vi "Init DMM - Voltage Mode.vi"(8 "error in (no error)":errorcluster, 9 "Switch -> DMM Trigger":u16, 10 "DMM -> Switch Trigger":u16, 11 "DMM Device in":refnum<k15>) -> (0 "error out":errorcluster, 3 "DMM Device out":refnum<k15>)   [LabVIEW 2011, in "Switch-DMM Custom Device.lvlib"]
uses:
  Switch-DMM Custom Device.lvlib
  <instrlib>/niDMM/nidmm.llb/niDMM Resolution in Digits.ctl
  <instrlib>/niDMM/nidmm.llb/niDMM Slope.ctl
  <instrlib>/niDMM/nidmm.llb/niDMM Sample Trigger.ctl
  <instrlib>/niDMM/nidmm.llb/niDMM Trigger.ctl
  <instrlib>/niDMM/nidmm.llb/niDMM Measurement Complete.ctl
  <instrlib>/niDMM/nidmm.llb/niDMM Function.ctl
  <instrlib>/niDMM/nidmm.llb/niDMM Configure Measurement Digits.vi
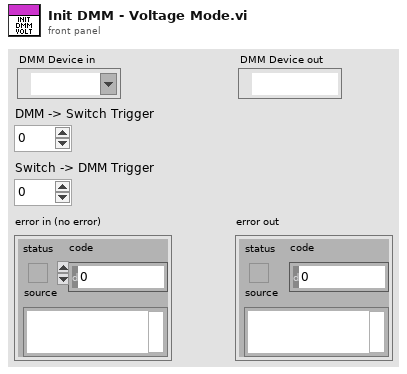
[diagram p1: front panel]
types:
  T1 = typedef "niDMM Sample Trigger.ctl" = enum16{"Immediate", "External", "TTL 0", "TTL 1", "TTL 2", "TTL 3", "TTL 4", "TTL 5", "TTL 6", "Interval", "Software", "TTL 7", "PXI Star", "LBR Trig 1", "Aux Trig 1"}
  T2 = typedef "niDMM Trigger.ctl" = enum16{"Immediate", "External", "TTL 0", "TTL 1", "TTL 2", "TTL 3", "TTL 4", "TTL 5", "TTL 6", "Software", "TTL 7", "PXI Star", "LBR Trig 1", "Aux Trig 1"}
  T3 = typedef "niDMM Measurement Complete.ctl" = enum16{"None", "External", "TTL 0", "TTL 1", "TTL 2", "TTL 3", "TTL 4", "TTL 5", "TTL 6", "TTL 7", "LBR Trig 0"}
  T4 = typedef "niDMM Function.ctl" = enum16{"DC Volts", "AC Volts", "DC Current", "AC Current", "2-wire Resistance", "4-wire Resistance", "Diode", "Frequency", "Period", "AC Volts DC Coupled", "Capacitance", "Inductance", "Temperature"}
  T5 = typedef "niDMM Resolution in Digits.ctl" = dbl
  T6 = typedef "niDMM Slope.ctl" = enum16{"Rising Edge", "Falling Edge"}
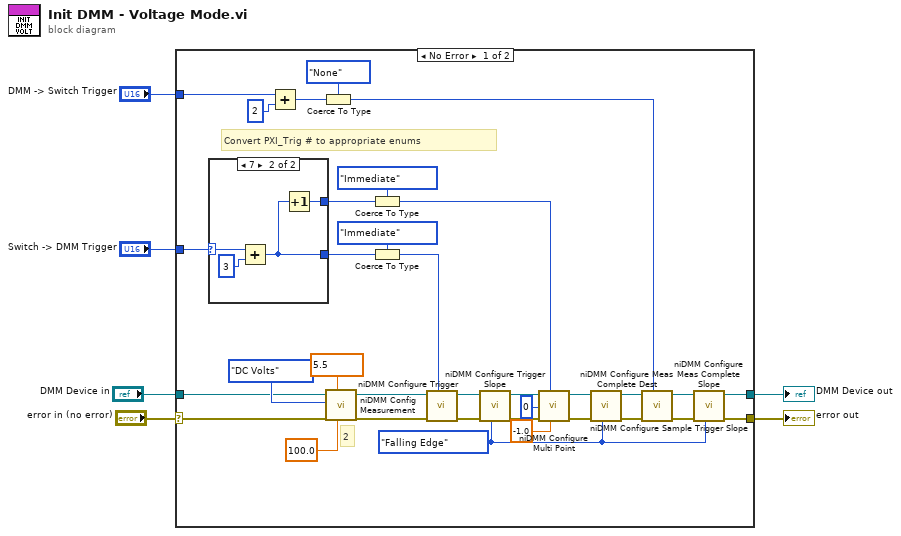
[diagram p0: block diagram]
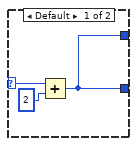
[diagram p2: hidden frame]
diagram:
  n1 = case shown="No Error" "error in (no error)" {
    selector: "error in (no error)" -> [w10 w48]
    tunnel: [w40 w49] -> w1
    tunnel: [w39 w48] -> w2
    tunnel: "DMM Device in" -> [w11 w49]
    tunnel: "DMM -> Switch Trigger" -> [w20 _]
    tunnel: "Switch -> DMM Trigger" -> [w18 _]
    frame No Error {
      w7 = T5 5.5 items=["3 1/2"=3.5, "4 1/2"=4.5, "5 1/2"=5.5, "6 1/2"=6.5, "7 1/2"=7.5] ("Resolution in Digits")
      w9 = niDMM_Slope."Falling Edge" ("Slope")
      # "Convert PXI_Trig # to appropriate enums"
      # "2"
      n2 = case shown="7" w18 {
        selector: w18 -> [w42 w46]
        tunnel: [w41 w45] -> w17
        tunnel: [w41 w44] -> w14
        frame Default {
          n3 = Add(x=w42, y=u16 2) -> (x+y=w41:u16)
        }
        frame 7 {
          n4 = Add(x=w46, y=u16 3) -> (x+y=w45:u16)
          n5 = Increment(x=w45) -> (x+1=w44:u16)
        }
      }
      n6 = Add(x=w20, y=u16 2) -> (x+y=w22:u16)
      n7 = Coerce To Type(0:w22, 1:niDMM_Measurement_Complete."None" ("Measurement Complete Destination")) -> (2:w19:T3)
      n8 = call-poly <instrlib>:"niDMM Config Measurement.vi"("Range"=100.0 ("range"), "Resolution in Digits"=w7, "error in (no error)"=w10, "Function"=niDMM_Function."DC Volts" ("measurement type"), "instrument handle"=w11) -> ("error out"=w24:errorcluster, "instrument handle out"=w25:refnum<k15>)  [unwired: 5 out]
      n9 = Coerce To Type(0:w14, 1:niDMM_Sample_Trigger."Immediate" ("Sample Trigger")) -> (2:w12:T1)
      n10 = Coerce To Type(0:w17, 1:niDMM_Trigger."Immediate" ("trigger source")) -> (2:w15:T2)
      n11 = call <instrlib>:"niDMM Configure Trigger.vi"("Trigger Source"=w15, "error in (no error)"=w24, "instrument handle"=w25) -> ("error out"=w37:errorcluster, "instrument handle out"=w38:refnum<k15>)  [unwired: 1 in, 6 out]
      n12 = call <instrlib>:"niDMM Configure Trigger Slope.vi"("Slope"=w9, "error in (no error)"=w37, "instrument handle"=w38) -> ("error out"=w35:errorcluster, "instrument handle out"=w36:refnum<k15>)  [unwired: 7 out]
      n13 = call <instrlib>:"niDMM Configure Multi Point.vi"("Sample Interval (sec)"=-1.0, "Sample Trigger"=w12, "error in (no error)"=w35, "Sample Count"=0 ("sample count"), "instrument handle"=w36) -> ("error out"=w33:errorcluster, "instrument handle out"=w34:refnum<k15>)  [unwired: 1 in, 4 out]
      n14 = call <instrlib>:"niDMM Configure Sample Trigger Slope.vi"("Slope"=w9, "error in (no error)"=w33, "instrument handle"=w34) -> ("error out"=w31:errorcluster, "instrument handle out"=w30:refnum<k15>)  [unwired: 7 out]
      n15 = call <instrlib>:"niDMM Configure Meas Complete Dest.vi"("Measurement Complete Destination"=w19, "error in (no error)"=w31, "instrument handle"=w30) -> ("error out"=w28:errorcluster, "instrument handle out"=w29:refnum<k15>)  [unwired: 7 out]
      n16 = call <instrlib>:"niDMM Configure Meas Complete Slope.vi"("Slope"=w9, "error in (no error)"=w28, "instrument handle"=w29) -> ("error out"=w39:errorcluster, "instrument handle out"=w40:refnum<k15>)  [unwired: 7 out]
    }
    frame Error {
    }
  }
  "DMM Device out" <- w1
  "error out" <- w2
